vi "LED2472G_Scrolling Text LED Matrix.vi"(8 "error in (no error)":errorcluster, 10 "Color Box":u32(colorbox) caption="Text color", 11 "String":string caption="Text to scroll") -> (0 "error out":errorcluster)   [LabVIEW 2020]
uses:
  <vilib>/MakerHub/LINX/Public/Utilities/Open Local.vi
  <vilib>/MakerHub/LINX/LMH-LINX.lvlib
  RPI_SenseHat/LED2472G/LED2472G/LED2472G.lvclass
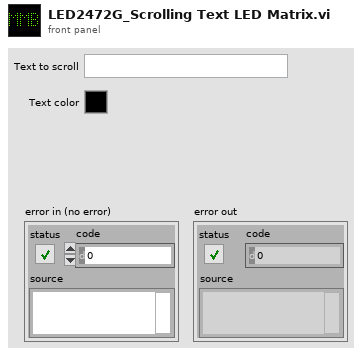
[diagram p1: front panel]
types:
  T1 = typedef "LMH-LINX.lvlib/LINX Ref.ctl" = cluster{"IO":T2, "Interface":T3, "LINX Device Config":T4}
  T2 = typedef "LMH-LINX.lvlib/Platform.ctl" = enum16{"Remote", "Local"}
  T3 = typedef "LMH-LINX.lvlib/Interface.ctl" = enum16{"Serial", "TCP"}
  T4 = typedef "LMH-LINX.lvlib/Device.lvlib/LINX Device Config.ctl" = cluster{"Interface":T3, "COM Port":refnum<visa-resource-name>, "TCP Configuration":T5, "Device Family":u8, "Device ID":u8, "Device Name":string, "TCP Ref":refnum<k5>, "Channels":T6}
  T5 = typedef "LMH-LINX.lvlib/Device.lvlib/TCP Config.ctl" = cluster{"IP Address":string, "Port":u16}
  T6 = typedef "LMH-LINX.lvlib/Channels.ctl" = cluster{"DI":u8[], "DO":u8[], "AI":u8[], "AO":u8[], "PWM":u8[], "QE":u8[], "UART":u8[], "I2C 2":u8[], "SPI":u8[], "CAN":u8[], "Servo":u8[], "AI Ref (V)":dbl, "AI Resolution (Bits)":u8, "AO Ref (V)":dbl, "AO Resolution (Bits)":u8}
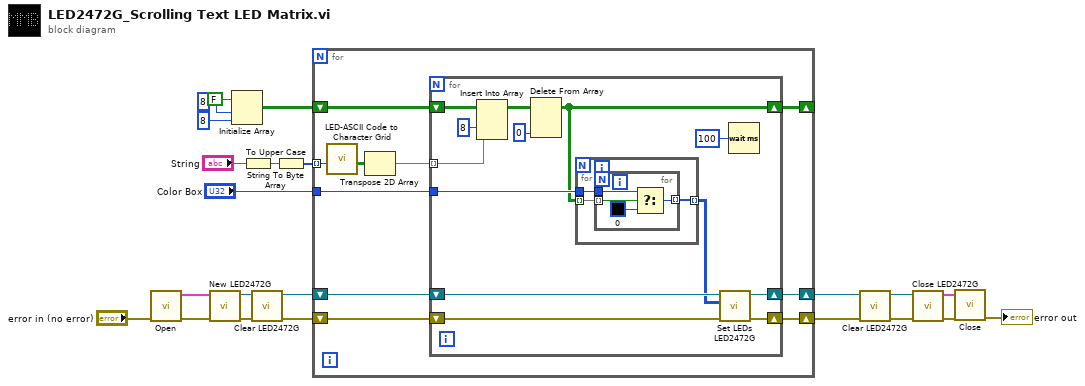
[diagram p0: block diagram]
diagram:
  n1 = call-poly <vilib>:"Open.vi"("Error In"="error in (no error)") -> ("Error Out"=w19:errorcluster, "LINX Resource"=w20:T1)  [unwired: 8 in, 1 out]
  n2 = call "New LED2472G.vi"("error in (no error)"=w19, "LINX Resource"=w20) -> ("error out"=w21:errorcluster, "LED2472G out"=w22:refnum<class "LED2472G.lvclass">)  [unwired: 8 in]
  n3 = Initialize Array(FALSE, 8 ("dimension size"), 8 ("dimension size")) -> (w12:bool[][])
  n4 = To Upper Case(1:"String") -> (0:w18:string)
  n5 = call "Clear LED2472G.vi"("error in (no error)"=w21, "LED2472G in"=w22) -> ("error out"=w4:errorcluster, "LED2472G out"=w10:refnum<class "LED2472G.lvclass">)  [unwired: 8 in]
  n6 = String To Byte Array(string=w18) -> (unsigned byte array=w16:u8[])
  n7 = for {
    tunnel: w16 -> [w32] mode=indexing
    shift-right: [w29] -> _
    shift-left: w12 -> [w30]
    tunnel: "Color Box" -> [w27]
    shift-right: [w25] -> w9
    shift-left: w10 -> [w26]
    shift-right: [w23] -> w3
    shift-left: w4 -> [w24]
    n8 = call "LED-ASCII Code to Character Grid.vi"("ASCII Value"=w32) -> ("Character Grid"=w31:bool[][])  [unwired: 10 in]
    n9 = Transpose 2D Array(2D array=w31) -> (transposed array=w28:bool[][])
    n10 = for {
      shift-right: [w36] -> w29
      shift-left: w30 -> [w44]
      tunnel: w28 -> [w43] mode=indexing
      tunnel: w27 -> [w42]
      shift-right: [w40] -> w25
      shift-left: w26 -> [w41]
      shift-right: [w33] -> w23
      shift-left: w24 -> [w34]
      n11 = Insert Into Array(array=w44, index (col)=8 ("disabled index (col)"), new element=w43) -> (w37:bool[][])  [unwired: 1 in]
      n12 = Delete From Array(array=w37, index (col)=0 ("disabled index (col)")) -> (array with subset deleted=w36:bool[][])  [unwired: 2 in, 1 out]
      n13 = for {
        tunnel: w36 -> [w48] mode=indexing
        tunnel: [w47] -> w39 mode=indexing
        tunnel: w42 -> [w46]
        n14 = for {
          tunnel: w48 -> [w52] mode=indexing
          tunnel: [w50] -> w47 mode=indexing
          tunnel: w46 -> [w49]
          n15 = Select(t=w49, s=w52, f=u32 0) -> (s? t:f=w50:u32)
        }
      }
      n16 = call "Set LEDs LED2472G.vi"("error in (no error)"=w34, "LED Matrix"=w39, "LED2472G in"=w41) -> ("error out"=w33:errorcluster, "LED2472G out"=w40:refnum<class "LED2472G.lvclass">)  [unwired: 7 in]
      n17 = Wait (ms)(milliseconds to wait=u32 100) -> ()  [unwired: 1 out]
    }
  }
  n18 = call "Clear LED2472G.vi"("error in (no error)"=w3, "LED2472G in"=w9) -> ("error out"=w5:errorcluster, "LED2472G out"=w8:refnum<class "LED2472G.lvclass">)  [unwired: 8 in]
  n19 = call "Close LED2472G.vi"("error in (no error)"=w5, "LED2472G in"=w8) -> ("error out"=w7:errorcluster, "LINX Resource"=w6:T1)  [unwired: 8 in]
  n20 = call <vilib>:"Close.vi"("Error In"=w7, "LINX Resource"=w6) -> ("Error Out"=→"error out":errorcluster)  [unwired: 9 in]
